vi "readBufferTest.vi"() -> ()   [LabVIEW 2016]
uses:
  ElectrometerConfiguration/Controls/com_conf.ctl
  ts_electrometeruserevents/Typedefs/termChar.ctl
  Electrometer/Electrometer.lvclass
  ElectrometerConfiguration/ElectrometerCOMConfiguration.lvclass
  ts_electrometeruserevents/Typedefs/ElectrometerTypedefs.lvlib
  ts_electrometeruserevents/ConfigurationTC/ConfigurationTypedefs/ConfigurationTypedefs.lvlib
panel:
  out "read buffer":string
  in  "Serial Communication":T1={"Baud Rate"=57600.0, "VISA resource name"="ASRL5::INSTR", "Parity"=0, "Data Bits"=8, "Stop Bits"=10, "Flow Control"=0, "termChar"=enum."LF"} {"Flow Control" items=["None", "XON/XOFF", "RTS/CTS", "XON/XOFF & RTS/CTS", "DTR/DSR", "XON/XOFF & DTR/DSR"]; "Stop Bits" items=["1.0"=10, "1.5"=15, "2.0"=20]; "Data Bits" items=["7"=7, "8"=8]; "Parity" items=["None", "Odd", "Even", "Mark", "Space"]}
  out "Error Message":string
  out "Error Code":i32[](array[numeric])
  out "Voltage":string
  out "error out":errorcluster
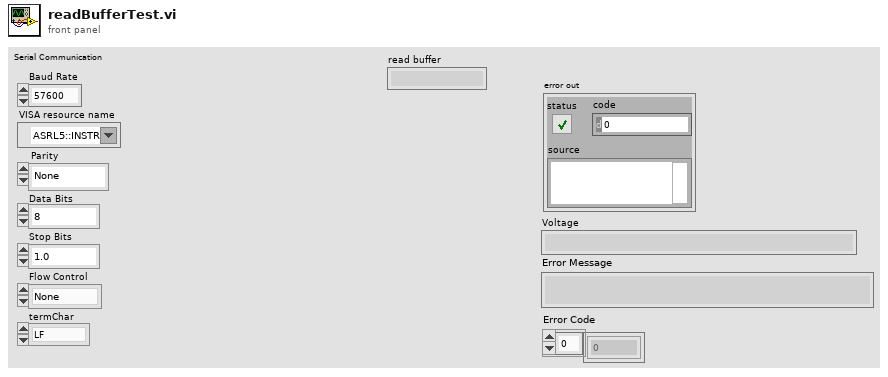
[diagram p1: front panel]
types:
  T1 = typedef "ConfigurationTypedefs.lvlib/com_conf.ctl" = cluster{"Baud Rate":dbl, "VISA resource name":refnum<visa-resource-name>, "Parity":u16, "Data Bits":u16, "Stop Bits":u16, "Flow Control":u16, "termChar":T2}
  T2 = typedef "ElectrometerTypedefs.lvlib/termChar.ctl" = enum16{"CR", "CR+LF", "LF", "LF+CR"}
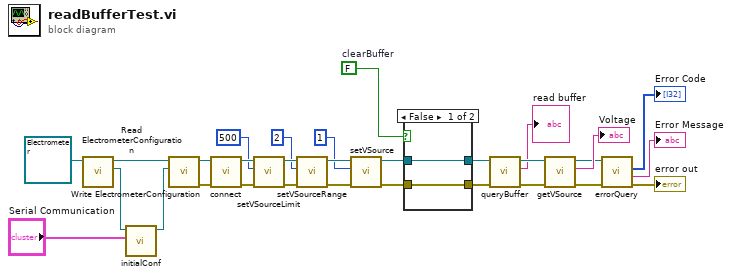
[diagram p0: block diagram]
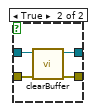
[diagram p2: hidden frame]
diagram:
  w1 = FALSE  # clearBuffer
  n1 = call "Read ElectrometerConfiguration.vi"("Electrometer in"=refnum<class "Electrometer.lvclass"> refnum ("Electrometer.lvclass")) -> ("ElectrometerConfiguration"=w28:refnum<class "ElectrometerCOMConfiguration.lvclass">, "Electrometer out"=w29:refnum<class "Electrometer.lvclass">)  [unwired: 8 in, 1 out]
  n2 = call "initialConf.vi"("Serial Communication"="Serial Communication", "ElectrometerConfiguration In"=w28) -> ("ElectrometerConfiguration Out"=w27:refnum<class "ElectrometerCOMConfiguration.lvclass">)  [unwired: 9 in]
  n3 = call-dynamic "Write ElectrometerConfiguration.vi"("ElectrometerConfiguration"=w27, "Electrometer in"=w29) -> ("error out"=w25:errorcluster, "Electrometer out"=w26:refnum<class "Electrometer.lvclass">)  [unwired: 8 in]
  n4 = call "connect.vi"("error in (no error)"=w25, "Electrometer in"=w26) -> ("error out"=w21:errorcluster, "Electrometer out"=w24:refnum<class "Electrometer.lvclass">)  [unwired: 7 in, 1 out]
  n5 = call "setVSourceLimit.vi"("error in (no error)"=w21, "Volt Limit"=500, "Electrometer in"=w24) -> ("error out"=w20:errorcluster, "Electrometer out"=w23:refnum<class "Electrometer.lvclass">)  [unwired: 7 in]
  n6 = call "setVSourceRange.vi"("error in (no error)"=w20, "Volt Range"=2, "Electrometer in"=w23) -> ("error out"=w19:errorcluster, "Electrometer out"=w22:refnum<class "Electrometer.lvclass">)  [unwired: 7 in]
  n7 = call "setVSource.vi"("error in (no error)"=w19, "Volt"=1, "Electrometer in"=w22) -> ("error out"=w8:errorcluster, "Electrometer out"=w7:refnum<class "Electrometer.lvclass">)  [unwired: 7 in]
  n8 = case shown="False" w1 {
    tunnel: w8 -> [w31 w36]
    tunnel: w7 -> [w32 w35]
    tunnel: [w32 w34] -> w6
    tunnel: [w31 w33] -> w5
    frame False {
    }
    frame True {
      n9 = call "clearBuffer.vi"("error in (no error)"=w36, "Electrometer in"=w35) -> ("error out"=w33:errorcluster, "Electrometer out"=w34:refnum<class "Electrometer.lvclass">)  [unwired: 8 in]
    }
  }
  n10 = call "queryBuffer.vi"("error in (no error)"=w5, "Electrometer in"=w6) -> ("error out"=w4:errorcluster, "read buffer"=→"read buffer":string, "Electrometer out"=w3:refnum<class "Electrometer.lvclass">)  [unwired: 7 in]
  n11 = call "getVSource.vi"("error in (no error)"=w4, "Electrometer in"=w3) -> ("error out"=w12:errorcluster, "Voltage"=→"Voltage":string, "Electrometer out"=w11:refnum<class "Electrometer.lvclass">)  [unwired: 7 in]
  n12 = call "errorQuery.vi"("error in (no error)"=w12, "Electrometer in"=w11) -> ("error out"=→"error out":errorcluster, "Error Message"=→"Error Message":string, "Device Error"=→"Error Code":i32[])  [unwired: 6 in, 1 out]
